vi "Acquisition Timer.vi"(11 "Start In":bool, 13 "Reset":bool) -> (4 "Timestamp":u64, 15 "Start Out":bool)   [LabVIEW 2014]
panel:
  # "Copyright 2014 Vidrio Technologies\nScanImage 5 software is licensed under the Apache License, Version 2.0 (the \"License\"); you may not use any files contained\nwithin the ScanImage 5 release except in compliance with the License. You may obtain a copy of the License at\n http://www.apache.org/licenses/LICENSE-2.0\nUnless required by applicable law or agreed to in writing, software distributed under the License is distributed on an\n\"AS IS\" BASIS, WITHOUT WARRANTIES OR CONDITIONS OF ANY KIND, either express or implied. See the License for the\n specific language governing permissions and limitations under the License."
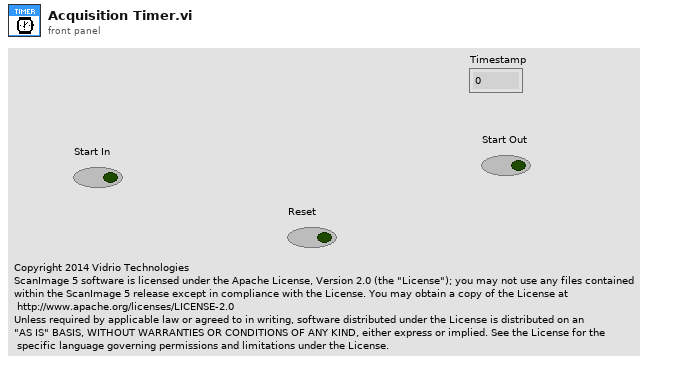
[diagram p1: front panel]
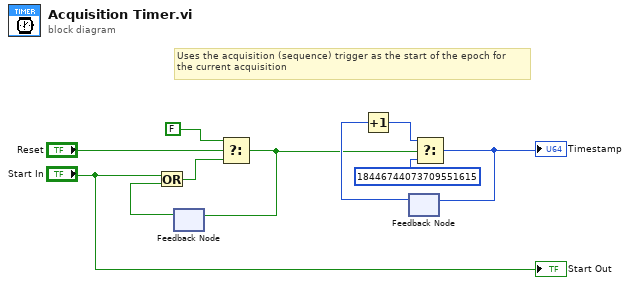
[diagram p0: block diagram]
diagram:
  # "Uses the acquisition (sequence) trigger as the start of the epoch for\nthe current acquisition"
  n1 = feedback #1() -> (w8:bool)  [unwired: 1 in]
  n2 = Or(x="Start In", y=w8) -> (x .or. y?=w5:bool)
  n3 = Select(t=FALSE ("Start"), s="Reset", f=w5) -> (s? t:f=w4:bool)
  n4 = feedback-in #1(w4) -> ()
  n5 = feedback #2() -> (w10:u64)  [unwired: 1 in]
  n6 = Increment(x=w10) -> (x+1=w3:u64)
  n7 = Select(t=w3, s=w4, f=u64 18446744073709551615) -> (s? t:f=w9:u64)
  "Timestamp" <- w9
  n8 = feedback-in #2(w9) -> ()
  "Start Out" <- "Start In"
